vi "Read Swipe Direction.vi"   [LabVIEW 2011, in "LMH-Leap.lvlib"]
doc: "Read swipe gesture directions (Up, Down, Left, Right, In, Out). Use the polymorphic instance to select between one or N swipe gestures."
uses:
  LMH-Leap.lvlib
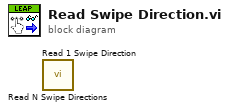
[diagram p0: block diagram]
diagram:
  n1 = call "Read N Swipe Directions.vi"() -> ()  [unwired: 8 in, 4 out]
  n2 = call "Read 1 Swipe Direction.vi"() -> ()  [unwired: 8 in, 4 out]
